vi "InitAPSxObject.vi"(8 "error in (no error)":errorcluster caption="错误输入（无错误）", 10 "AsicType":T1(ring), 11 "hASIC":i32) -> (0 "error out":errorcluster caption="错误输出", 1 "Message":string, 3 "hASIC out":i32)   [LabVIEW 2018]
doc: "该模板用于创建子VI。"
uses:
  APSx.dll/APSx.dll
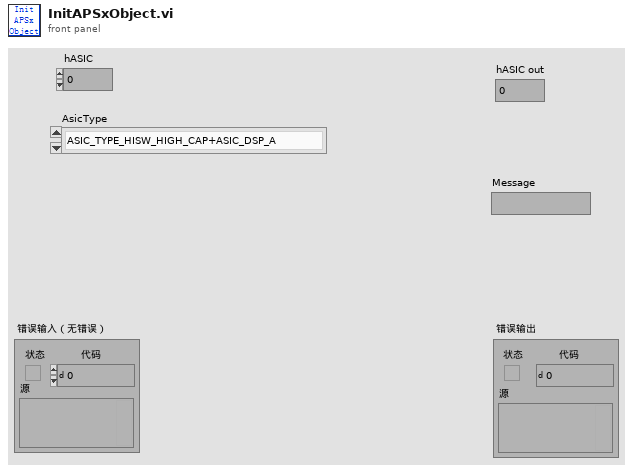
[diagram p1: front panel]
types:
  T1 = enum16{"ASIC_TYPE_HISW_HIGH_CAP+ASIC_DSP_A", "ASIC_TYPE_HISW_HIGH_CAP+ASIC_DSP_B"}
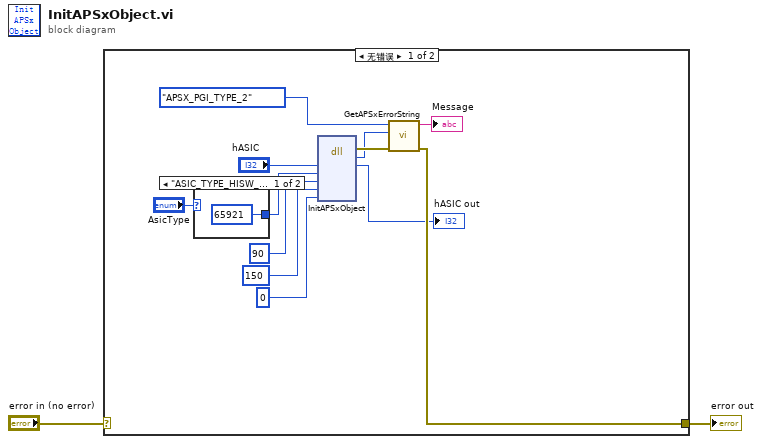
[diagram p0: block diagram]
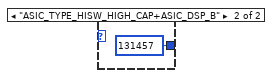
[diagram p2: hidden frame]
diagram:
  n1 = case shown="无错误" "error in (no error)" {
    selector: "error in (no error)" -> [_ w17]
    tunnel: [w5 w17] -> w1
    frame No Error {
      n2 = case shown="\"ASIC_TYPE_HISW_HIGH_CAP+ASIC_DSP_A\", 默认" "AsicType" {
        tunnel: [65921 ("AsicType") 131457 ("AsicType")] -> w13
        frame "ASIC_TYPE_HISW_HIGH_CAP+ASIC_DSP_A", Default {
        }
        frame "ASIC_TYPE_HISW_HIGH_CAP+ASIC_DSP_B" {
        }
      }
      n3 = dll-call lib="PTH2]abs D项目Feng恒隆项目Labview传感器对中台SourcesAPSx.dllAPSx.dll" fn="InitAPSxObject"("hASIC"="hASIC", "AsicType"=w13, "MaxOutCurrent"=90, "MaxOTPCurrent"=150, "OTPOffset"=0) -> (error out=w8:errorcluster, "Code"=w6:i32, "hASIC"=→"hASIC out":i32)  [unwired: 7 in, 1 out]
      n4 = call "GetAPSxErrorString.vi"("error in (no error)"=w8, "ErrorCode"=w6, "PGIType"=enum16{"APSX_PGI_TYPE_1", "APSX_PGI_TYPE_2"}."APSX_PGI_TYPE_2") -> ("error out"=w5:errorcluster, "Message"=→"Message":string)  [unwired: 7 in]
    }
    frame Error {
    }
  }
  "error out" <- w1
